vi "S4GUI_003.vi"(7 "Tab ObsEng":enum32{"Obs", "CCD modes", "Guider", "Eng"}(tab)) -> ()   [LabVIEW 2018] (continued)
                n2221 = call-dynamic "Get CCD_Config.vi"("error in (no error)"=w4421, "Interface in"=w4422) -> ("error out"=w4419:errorcluster, "output cluster"=w4418:T31, "Interface out"=w4423:refnum<class "Interface.lvclass">)  [unwired: 7 in]
                n2222 = Bundle By Name(cluster=w4418, "TRIGGER_MODE"=w4406) -> (w4420:T31)
                n2223 = call-dynamic "Set CCD_Config.vi"("error in (no error)"=w4419, "input cluster"=w4420, "Interface in"=w4423) -> ("error out"=w4417:errorcluster, "Interface out"=w4424:refnum<class "Interface.lvclass">)  [unwired: 7 in]
                n2224 = Flatten To String(anything=w4420, error in (no error)=w4417) -> (data string=w4415:string, error out=w4416:errorcluster)  [unwired: 2 in, 1 out]
                n2225 = call "Write flatted cluster.vi"("error in (no error)"=w4416, "flatted cluster"=w4415, "Interface in"=w4424) -> ("error out"=w4426:errorcluster, "Interface out"=w4425:refnum<class "Interface.lvclass">)  [unwired: 7 in]
                n2226 = call-dynamic "Write Interface.vi"("error in (no error)"=w4426, "Interface.lvclass"=w4425, "Channel in"=w4411) -> ("error out"=w4432:errorcluster, "Channel out"=w4433:refnum<class "Channel.lvclass">)  [unwired: 7 in]
                n2227 = call "Write section_name.vi"("error in (no error)"=w4432, "section_name"="CCD_ACS3", "Channel in"=w4433) -> ("error out"=w4430:errorcluster, "Channel out"=w4436:refnum<class "Channel.lvclass">)  [unwired: 7 in]
                n2228 = call-dynamic "save config.vi"("error in (no error)"=w4430, "file config"="lastsaved.cfg", "Channel in"=w4436) -> ("error out"=w4431:errorcluster, "Channel out"=w4437:refnum<class "Channel.lvclass">)  [unwired: 7 in]
                n2229 = call-dynamic "Read State Machine.vi"("error in (no error)"=w4431, "Device in"=w4437) -> ("error out"=w4427:errorcluster, "State Machine.lvclass"=w4439:refnum<class "State Machine.lvclass">, "Device out"=w4438:refnum<class "Channel.lvclass">)  [unwired: 7 in]
                n2230 = call-dynamic "Write State.vi"("error in (no error)"=w4427, "State"=60, "State Machine in"=w4439) -> ("error out"=w4428:errorcluster, "State Machine out"=w4440:refnum<class "State Machine.lvclass">)  [unwired: 7 in]
                n2231 = call-dynamic "Write State Machine.vi"("error in (no error)"=w4428, "State Machine.lvclass"=w4440, "Device in"=w4438) -> ("error out"=w4404:errorcluster, "Device out"=w4405:refnum<class "Channel.lvclass">)  [unwired: 7 in]
                n2232 = call-dynamic "Read prev ciclos.vi"("error in (no error)"=w4404, "Channel in"=w4405) -> ("error out"=w4402:errorcluster, "prev ciclos"=w4400:u32, "Channel out"=w4403:refnum<class "Channel.lvclass">)  [unwired: 7 in]
                n2233 = local write "#cycles ch3"(w4400) -> ()
                n2234 = property on="Cycles Done ch3" class="Slide (strict)"("Scale.Maximum"=w4400, "Scale.Minimum"=0.0 ("Scale.Range:Minimum")) -> ()  [unwired: 2 in, 2 out]
                n2235 = call-dynamic "Write Channel.vi"("error in (no error)"=w4402, "Channel.lvclass"=w4403, "Acquisition in"=w4412) -> ("error out"=w4407:errorcluster, "Acquisition out"=w4408:refnum<class "Acquisition.lvclass">)  [unwired: 7 in]
              }
            }
            n2236 = case shown="True" w4337 {
              tunnel: w4339 -> [w4356 w4367]
              tunnel: w4338 -> [w4355 w4366]
              tunnel: [w4356 w4365] -> w4310
              tunnel: [w4355 w4364] -> w4309
              tunnel: w4307 -> [_ w4363]
              frame False {
              }
              frame True {
                # "nome do arquivo .cfg"
                # "seção no arquivo .cfg"
                n2237 = call-dynamic "Read Channel.vi"("error in (no error)"=w4366, "Acquisition in"=w4367) -> ("error out"=w4394:errorcluster, "Channel.lvclass"=w4395:refnum<class "Channel.lvclass">, "Acquisition out"=w4396:refnum<class "Acquisition.lvclass">)  [unwired: 7 in]
                n2238 = call-dynamic "Read Interface.vi"("error in (no error)"=w4394, "Channel in"=w4395) -> ("error out"=w4387:errorcluster, "Interface.lvclass"=w4386:refnum<class "Interface.lvclass">, "Channel out"=w4397:refnum<class "Channel.lvclass">)  [unwired: 7 in]
                n2239 = call-dynamic "Get CCD_Config.vi"("error in (no error)"=w4387, "Interface in"=w4386) -> ("error out"=w4389:errorcluster, "output cluster"=w4390:T31, "Interface out"=w4385:refnum<class "Interface.lvclass">)  [unwired: 7 in]
                n2240 = Bundle By Name(cluster=w4390, "TRIGGER_MODE"=w4363) -> (w4388:T31)
                n2241 = call-dynamic "Set CCD_Config.vi"("error in (no error)"=w4389, "input cluster"=w4388, "Interface in"=w4385) -> ("error out"=w4391:errorcluster, "Interface out"=w4384:refnum<class "Interface.lvclass">)  [unwired: 7 in]
                n2242 = Flatten To String(anything=w4388, error in (no error)=w4391) -> (data string=w4393:string, error out=w4392:errorcluster)  [unwired: 2 in, 1 out]
                n2243 = call "Write flatted cluster.vi"("error in (no error)"=w4392, "flatted cluster"=w4393, "Interface in"=w4384) -> ("error out"=w4382:errorcluster, "Interface out"=w4383:refnum<class "Interface.lvclass">)  [unwired: 7 in]
                n2244 = call-dynamic "Write Interface.vi"("error in (no error)"=w4382, "Interface.lvclass"=w4383, "Channel in"=w4397) -> ("error out"=w4376:errorcluster, "Channel out"=w4375:refnum<class "Channel.lvclass">)  [unwired: 7 in]
                n2245 = call "Write section_name.vi"("error in (no error)"=w4376, "section_name"="CCD_ACS4", "Channel in"=w4375) -> ("error out"=w4378:errorcluster, "Channel out"=w4372:refnum<class "Channel.lvclass">)  [unwired: 7 in]
                n2246 = call-dynamic "save config.vi"("error in (no error)"=w4378, "file config"="lastsaved.cfg", "Channel in"=w4372) -> ("error out"=w4377:errorcluster, "Channel out"=w4371:refnum<class "Channel.lvclass">)  [unwired: 7 in]
                n2247 = call-dynamic "Read State Machine.vi"("error in (no error)"=w4377, "Device in"=w4371) -> ("error out"=w4381:errorcluster, "State Machine.lvclass"=w4369:refnum<class "State Machine.lvclass">, "Device out"=w4370:refnum<class "Channel.lvclass">)  [unwired: 7 in]
                n2248 = call-dynamic "Write State.vi"("error in (no error)"=w4381, "State"=60, "State Machine in"=w4369) -> ("error out"=w4380:errorcluster, "State Machine out"=w4368:refnum<class "State Machine.lvclass">)  [unwired: 7 in]
                n2249 = call-dynamic "Write State Machine.vi"("error in (no error)"=w4380, "State Machine.lvclass"=w4368, "Device in"=w4370) -> ("error out"=w4361:errorcluster, "Device out"=w4362:refnum<class "Channel.lvclass">)  [unwired: 7 in]
                n2250 = call-dynamic "Read prev ciclos.vi"("error in (no error)"=w4361, "Channel in"=w4362) -> ("error out"=w4359:errorcluster, "prev ciclos"=w4357:u32, "Channel out"=w4360:refnum<class "Channel.lvclass">)  [unwired: 7 in]
                n2251 = local write "#cycles ch4"(w4357) -> ()
                n2252 = property on="Cycles Done ch4" class="Slide (strict)"("Scale.Maximum"=w4357, "Scale.Minimum"=0.0 ("Scale.Range:Minimum")) -> ()  [unwired: 2 in, 2 out]
                n2253 = call-dynamic "Write Channel.vi"("error in (no error)"=w4359, "Channel.lvclass"=w4360, "Acquisition in"=w4396) -> ("error out"=w4364:errorcluster, "Acquisition out"=w4365:refnum<class "Acquisition.lvclass">)  [unwired: 7 in]
              }
            }
            n2254 = case shown="True" w4343 {
              tunnel: w4345 -> [w4442 w4453]
              tunnel: w4344 -> [w4441 w4452]
              tunnel: [w4442 w4451] -> w4314
              tunnel: [w4441 w4450] -> w4313
              tunnel: w4307 -> [_ w4449]
              frame False {
              }
              frame True {
                # "nome do arquivo .cfg"
                # "seção no arquivo .cfg"
                n2255 = call-dynamic "Read Channel.vi"("error in (no error)"=w4452, "Acquisition in"=w4453) -> ("error out"=w4457:errorcluster, "Channel.lvclass"=w4456:refnum<class "Channel.lvclass">, "Acquisition out"=w4455:refnum<class "Acquisition.lvclass">)  [unwired: 7 in]
                n2256 = call-dynamic "Read Interface.vi"("error in (no error)"=w4457, "Channel in"=w4456) -> ("error out"=w4464:errorcluster, "Interface.lvclass"=w4465:refnum<class "Interface.lvclass">, "Channel out"=w4454:refnum<class "Channel.lvclass">)  [unwired: 7 in]
                n2257 = call-dynamic "Get CCD_Config.vi"("error in (no error)"=w4464, "Interface in"=w4465) -> ("error out"=w4462:errorcluster, "output cluster"=w4461:T31, "Interface out"=w4466:refnum<class "Interface.lvclass">)  [unwired: 7 in]
                n2258 = Bundle By Name(cluster=w4461, "TRIGGER_MODE"=w4449) -> (w4463:T31)
                n2259 = call-dynamic "Set CCD_Config.vi"("error in (no error)"=w4462, "input cluster"=w4463, "Interface in"=w4466) -> ("error out"=w4460:errorcluster, "Interface out"=w4467:refnum<class "Interface.lvclass">)  [unwired: 7 in]
                n2260 = Flatten To String(anything=w4463, error in (no error)=w4460) -> (data string=w4458:string, error out=w4459:errorcluster)  [unwired: 2 in, 1 out]
                n2261 = call "Write flatted cluster.vi"("error in (no error)"=w4459, "flatted cluster"=w4458, "Interface in"=w4467) -> ("error out"=w4469:errorcluster, "Interface out"=w4468:refnum<class "Interface.lvclass">)  [unwired: 7 in]
                n2262 = call-dynamic "Write Interface.vi"("error in (no error)"=w4469, "Interface.lvclass"=w4468, "Channel in"=w4454) -> ("error out"=w4475:errorcluster, "Channel out"=w4476:refnum<class "Channel.lvclass">)  [unwired: 7 in]
                n2263 = call "Write section_name.vi"("error in (no error)"=w4475, "section_name"="CCD_ACS2", "Channel in"=w4476) -> ("error out"=w4473:errorcluster, "Channel out"=w4479:refnum<class "Channel.lvclass">)  [unwired: 7 in]
                n2264 = call-dynamic "save config.vi"("error in (no error)"=w4473, "file config"="lastsaved.cfg", "Channel in"=w4479) -> ("error out"=w4474:errorcluster, "Channel out"=w4480:refnum<class "Channel.lvclass">)  [unwired: 7 in]
                n2265 = call-dynamic "Read State Machine.vi"("error in (no error)"=w4474, "Device in"=w4480) -> ("error out"=w4470:errorcluster, "State Machine.lvclass"=w4482:refnum<class "State Machine.lvclass">, "Device out"=w4481:refnum<class "Channel.lvclass">)  [unwired: 7 in]
                n2266 = call-dynamic "Write State.vi"("error in (no error)"=w4470, "State"=60, "State Machine in"=w4482) -> ("error out"=w4471:errorcluster, "State Machine out"=w4483:refnum<class "State Machine.lvclass">)  [unwired: 7 in]
                n2267 = call-dynamic "Write State Machine.vi"("error in (no error)"=w4471, "State Machine.lvclass"=w4483, "Device in"=w4481) -> ("error out"=w4447:errorcluster, "Device out"=w4448:refnum<class "Channel.lvclass">)  [unwired: 7 in]
                n2268 = call-dynamic "Read prev ciclos.vi"("error in (no error)"=w4447, "Channel in"=w4448) -> ("error out"=w4445:errorcluster, "prev ciclos"=w4443:u32, "Channel out"=w4446:refnum<class "Channel.lvclass">)  [unwired: 7 in]
                n2269 = local write "#cycles ch2"(w4443) -> ()
                n2270 = property on="Cycles Done ch2" class="Slide (strict)"("Scale.Maximum"=w4443, "Scale.Minimum"=0.0 ("Scale.Range:Minimum")) -> ()  [unwired: 2 in, 2 out]
                n2271 = call-dynamic "Write Channel.vi"("error in (no error)"=w4445, "Channel.lvclass"=w4446, "Acquisition in"=w4455) -> ("error out"=w4450:errorcluster, "Acquisition out"=w4451:refnum<class "Acquisition.lvclass">)  [unwired: 7 in]
              }
            }
            n2272 = case shown="True" w4346 {
              tunnel: [w4484 w4522] -> w4315
              tunnel: [w4485 w4521] -> w4316
              tunnel: w4348 -> [w4485 w4494]
              tunnel: w4347 -> [w4484 w4493]
              tunnel: w4307 -> [_ w4492]
              frame False {
              }
              frame True {
                # "nome do arquivo .cfg"
                # "seção no arquivo .cfg"
                n2273 = call-dynamic "Read Channel.vi"("error in (no error)"=w4493, "Acquisition in"=w4494) -> ("error out"=w4523:errorcluster, "Channel.lvclass"=w4524:refnum<class "Channel.lvclass">, "Acquisition out"=w4525:refnum<class "Acquisition.lvclass">)  [unwired: 7 in]
                n2274 = call-dynamic "Read Interface.vi"("error in (no error)"=w4523, "Channel in"=w4524) -> ("error out"=w4514:errorcluster, "Interface.lvclass"=w4513:refnum<class "Interface.lvclass">, "Channel out"=w4526:refnum<class "Channel.lvclass">)  [unwired: 7 in]
                n2275 = call-dynamic "Get CCD_Config.vi"("error in (no error)"=w4514, "Interface in"=w4513) -> ("error out"=w4516:errorcluster, "output cluster"=w4517:T31, "Interface out"=w4512:refnum<class "Interface.lvclass">)  [unwired: 7 in]
                n2276 = Bundle By Name(cluster=w4517, "TRIGGER_MODE"=w4492) -> (w4515:T31)
                n2277 = call-dynamic "Set CCD_Config.vi"("error in (no error)"=w4516, "input cluster"=w4515, "Interface in"=w4512) -> ("error out"=w4518:errorcluster, "Interface out"=w4511:refnum<class "Interface.lvclass">)  [unwired: 7 in]
                n2278 = Flatten To String(anything=w4515, error in (no error)=w4518) -> (data string=w4520:string, error out=w4519:errorcluster)  [unwired: 2 in, 1 out]
                n2279 = call "Write flatted cluster.vi"("error in (no error)"=w4519, "flatted cluster"=w4520, "Interface in"=w4511) -> ("error out"=w4509:errorcluster, "Interface out"=w4510:refnum<class "Interface.lvclass">)  [unwired: 7 in]
                n2280 = call-dynamic "Write Interface.vi"("error in (no error)"=w4509, "Interface.lvclass"=w4510, "Channel in"=w4526) -> ("error out"=w4504:errorcluster, "Channel out"=w4503:refnum<class "Channel.lvclass">)  [unwired: 7 in]
                n2281 = call "Write section_name.vi"("error in (no error)"=w4504, "section_name"="CCD_ACS1", "Channel in"=w4503) -> ("error out"=w4505:errorcluster, "Channel out"=w4500:refnum<class "Channel.lvclass">)  [unwired: 7 in]
                n2282 = call-dynamic "save config.vi"("error in (no error)"=w4505, "file config"="lastsaved.cfg", "Channel in"=w4500) -> ("error out"=w4495:errorcluster, "Channel out"=w4496:refnum<class "Channel.lvclass">)  [unwired: 7 in]
                n2283 = call-dynamic "Read State Machine.vi"("error in (no error)"=w4495, "Device in"=w4496) -> ("error out"=w4508:errorcluster, "State Machine.lvclass"=w4498:refnum<class "State Machine.lvclass">, "Device out"=w4499:refnum<class "Channel.lvclass">)  [unwired: 7 in]
                n2284 = call-dynamic "Write State.vi"("error in (no error)"=w4508, "State"=60, "State Machine in"=w4498) -> ("error out"=w4507:errorcluster, "State Machine out"=w4497:refnum<class "State Machine.lvclass">)  [unwired: 7 in]
                n2285 = call-dynamic "Write State Machine.vi"("error in (no error)"=w4507, "State Machine.lvclass"=w4497, "Device in"=w4499) -> ("error out"=w4490:errorcluster, "Device out"=w4491:refnum<class "Channel.lvclass">)  [unwired: 7 in]
                n2286 = call-dynamic "Read prev ciclos.vi"("error in (no error)"=w4490, "Channel in"=w4491) -> ("error out"=w4488:errorcluster, "prev ciclos"=w4486:u32, "Channel out"=w4489:refnum<class "Channel.lvclass">)  [unwired: 7 in]
                n2287 = local write "#cycles ch1"(w4486) -> ()
                n2288 = property on="Cycles Done ch1" class="Slide (strict)"("Scale.Maximum"=w4486, "Scale.Minimum"=0.0 ("Scale.Range:Minimum")) -> ()  [unwired: 2 in, 2 out]
                n2289 = call-dynamic "Write Channel.vi"("error in (no error)"=w4488, "Channel.lvclass"=w4489, "Acquisition in"=w4525) -> ("error out"=w4522:errorcluster, "Acquisition out"=w4521:refnum<class "Acquisition.lvclass">)  [unwired: 7 in]
              }
            }
            n2290 = call-dynamic "Write AcquisitionA.vi"("error in (no error)"=w4315, "Acquisition.lvclass"=w4316, "S4ACS_GUI in"=w4317) -> ("error out"=w4323:errorcluster, "S4ACS_GUI out"=w4326:refnum<class "S4GUI.lvclass">)  [unwired: 7 in]
            n2291 = call "Write AcquisitionB.vi"("error in (no error)"=w4313, "Acquisition.lvclass"=w4314, "S4ACS_GUI in"=w4326) -> ("error out"=w4322:errorcluster, "S4ACS_GUI out"=w4325:refnum<class "S4GUI.lvclass">)  [unwired: 7 in]
            n2292 = call-dynamic "Write AcquisitionC.vi"("error in (no error)"=w4311, "Acquisition.lvclass"=w4312, "S4ACS_GUI in"=w4325) -> ("error out"=w4321:errorcluster, "S4ACS_GUI out"=w4324:refnum<class "S4GUI.lvclass">)  [unwired: 7 in]
            n2293 = call-dynamic "Write AcquisitionD.vi"("error in (no error)"=w4309, "Acquisition.lvclass"=w4310, "S4ACS_GUI in"=w4324) -> ("error out"=w4320:errorcluster, "S4ACS_GUI out"=w4319:refnum<class "S4GUI.lvclass">)  [unwired: 7 in]
            n2294 = Merge Errors(w4323, w4322, w4321, w4320) -> (w4318:errorcluster)
          }
        }
        n2295 = Concatenate Strings(w4071, " MODE SELECTED" ("User Event")) -> (w4076:string)
        n2296 = call-dynamic "Write sync.vi"("error in (no error)"=w4089, "sync"=w4091, "S4ACS_GUI in"=w4090) -> ("error out"=w4074:errorcluster, "S4ACS_GUI out"=w4075:refnum<class "S4GUI.lvclass">)  [unwired: 7 in]
        n2297 = call-dynamic "Write User Event.vi"("error in (no error)"=w4074, "User Event"=w4076, "S4GUI in"=w4075) -> ("error out"=w4072:errorcluster, "S4GUI out"=w4073:refnum<class "S4GUI.lvclass">)  [unwired: 7 in]
      }
      event "SendExpose": Value Change {
        n2298 = event-data() -> ("NewVal"=w4527:bool)  [unwired: 1 in]
        n2299 = disable-structure shown="Enabled" {
          disable-tunnel: w4527 -> [w4665 w4666]
          disable-tunnel: [w4664 w4666] -> w4528
          frame Disabled {
            n2300 = Not(x=w4665) -> (.not. x?=w4664:bool)
          }
          frame Enabled {
          }
        }
        n2301 = disable-structure shown="Enabled" {
          disable-tunnel: w4612 -> [w4627 w4663]
          disable-tunnel: w4611 -> [w4618 w4662]
          disable-tunnel: [w4615 w4663] -> w4530
          disable-tunnel: [w4614 w4662] -> w4529
          disable-tunnel: w4527 -> [w4613 _]
          frame Disabled {
            n2302 = call-dynamic "Read Sync Box.lvclass.vi"("error in (no error)"=w4618, "SPARC4_AC in"=w4627) -> ("error out"=w4620:errorcluster, "Sync Box.lvclass"=w4626:refnum<class "Sync Box.lvclass">, "SPARC4_AC out"=w4623:refnum<class "S4GUI.lvclass">)  [unwired: 7 in]
            n2303 = call-dynamic "Read Stream.vi"("error in (no error)"=w4620, "Server in"=w4626) -> ("error out"=w4619:errorcluster, "Stream.lvclass"=w4628:refnum<class "Stream.lvclass">, "Server out"=w4617:refnum<class "Sync Box.lvclass">)  [unwired: 7 in]
            n2304 = case shown="True" w4613 {
              tunnel: [w4631 w4648] -> w4621
              tunnel: w4628 -> [w4633 w4638]
              tunnel: [w4632 w4644] -> w4625
              tunnel: w4619 -> [w4630 w4636]
              tunnel: w4617 -> [w4629 w4637]
              tunnel: [w4629 w4637] -> w4616
              frame False {
                n2305 = call-dynamic "End.vi"("error in (no error)"=w4630, "Stream in"=w4633) -> ("error out"=w4631:errorcluster, "Stream out"=w4632:refnum<class "Stream.lvclass">)  [unwired: 8 in]
              }
              frame True {
                w4641 = errorcluster {"status"=FALSE, "code"=0, "source"=""} ("error in (no error)")
                w4659 = FALSE ("Wait Until Done")
                w4654 = FALSE ("Wait Until Done")
                n2306 = call-dynamic "Read comfile name1.vi"("error in (no error)"=w4636, "Stream in"=w4638) -> ("error out"=w4650:errorcluster, "comfile name1"=w4651:string, "Stream out"=w4647:refnum<class "Stream.lvclass">)  [unwired: 7 in]
                n2307 = call <vilib>:"Application Directory.vi"() -> ("Application Directory"=w4656:path)
                n2308 = call <vilib>:"Application Directory.vi"() -> ("Application Directory"=w4660:path)
                n2309 = Build Path(base path=w4660, name or relative path=w4651) -> (appended path=w4661:path)
                n2310 = Open VI Reference(vi path=w4661, error in (no error)=w4650) -> (vi reference=w4653:refnum<vi>, error out=w4652:errorcluster)  [unwired: 4 in]
                n2311 = invoke class="VI" method="Run VI"(reference=w4653, error in=w4652, "Wait until done"=w4654, "Auto Dispose Ref"=w4654) -> (reference out=w4643:refnum<vi>, error out=→"error out 7":errorcluster)  [unwired: 1 in, 3 out]
                n2312 = call-dynamic "Write commfile ref1.vi"("error in (no error)"=w4641, "commfile ref1"=w4643, "Stream in"=w4647) -> ("error out"=w4635:errorcluster, "Stream out"=w4646:refnum<class "Stream.lvclass">)  [unwired: 7 in]
                n2313 = call-dynamic "Read comfile name2.vi"("error in (no error)"=w4635, "Stream in"=w4646) -> ("error out"=w4634:errorcluster, "comfile name2"=w4649:string, "Stream out"=w4645:refnum<class "Stream.lvclass">)  [unwired: 7 in]
                n2314 = Build Path(base path=w4656, name or relative path=w4649) -> (appended path=w4655:path)
                n2315 = Open VI Reference(vi path=w4655, error in (no error)=w4634) -> (vi reference=w4657:refnum<vi>, error out=w4658:errorcluster)  [unwired: 4 in]
                n2316 = invoke class="VI" method="Run VI"(reference=w4657, error in=w4658, "Wait until done"=w4659, "Auto Dispose Ref"=w4659) -> (reference out=w4642:refnum<vi>, error out=→"error out 8":errorcluster)  [unwired: 1 in, 3 out]
                n2317 = call-dynamic "Write commfile ref2.vi"("error in (no error)"=w4641, "commfile ref2"=w4642, "Stream in"=w4645) -> ("error out"=w4648:errorcluster, "Stream out"=w4644:refnum<class "Stream.lvclass">)  [unwired: 7 in]
              }
            }
            n2318 = call-dynamic "Write Stream.vi"("error in (no error)"=w4621, "Stream.lvclass"=w4625, "Server in"=w4616) -> ("error out"=w4622:errorcluster, "Server out"=w4624:refnum<class "Sync Box.lvclass">)  [unwired: 7 in]
            n2319 = call-dynamic "Write Sync Box.lvclass.vi"("error in (no error)"=w4622, "Sync Box.lvclass"=w4624, "SPARC4_AC in"=w4623) -> ("error out"=w4614:errorcluster, "SPARC4_AC out"=w4615:refnum<class "S4GUI.lvclass">)  [unwired: 7 in]
          }
          frame Enabled {
          }
        }
        n2320 = call-dynamic "Read AcquisitionC.vi"("error in (no error)"=w4529, "S4ACS_GUI in"=w4530) -> ("error out"=w4554:errorcluster, "Acquisition.lvclass"=w4555:refnum<class "Acquisition.lvclass">)  [unwired: 7 in, 1 out]
        n2321 = call-dynamic "Read AcquisitionA.vi"("error in (no error)"=w4529, "S4ACS_GUI in"=w4530) -> ("error out"=w4591:errorcluster, "Acquisition.lvclass"=w4590:refnum<class "Acquisition.lvclass">, "S4ACS_GUI out"=w4607:refnum<class "S4GUI.lvclass">)  [unwired: 7 in]
        n2322 = call "Read AcquisitionB.vi"("error in (no error)"=w4529, "S4ACS_GUI in"=w4530) -> ("error out"=w4571:errorcluster, "Acquisition.lvclass"=w4572:refnum<class "Acquisition.lvclass">)  [unwired: 7 in, 1 out]
        n2323 = call-dynamic "Read AcquisitionD.vi"("error in (no error)"=w4529, "S4ACS_GUI in"=w4530) -> ("error out"=w4537:errorcluster, "Acquisition.lvclass"=w4538:refnum<class "Acquisition.lvclass">)  [unwired: 7 in, 1 out]
        n2324 = call-dynamic "Read Channel.vi"("error in (no error)"=w4537, "Acquisition in"=w4538) -> ("error out"=w4540:errorcluster, "Channel.lvclass"=w4542:refnum<class "Channel.lvclass">, "Acquisition out"=w4551:refnum<class "Acquisition.lvclass">)  [unwired: 7 in]
        n2325 = call-dynamic "Read Channel.vi"("error in (no error)"=w4554, "Acquisition in"=w4555) -> ("error out"=w4557:errorcluster, "Channel.lvclass"=w4559:refnum<class "Channel.lvclass">, "Acquisition out"=w4568:refnum<class "Acquisition.lvclass">)  [unwired: 7 in]
        n2326 = call-dynamic "Read Channel.vi"("error in (no error)"=w4571, "Acquisition in"=w4572) -> ("error out"=w4574:errorcluster, "Channel.lvclass"=w4576:refnum<class "Channel.lvclass">, "Acquisition out"=w4585:refnum<class "Acquisition.lvclass">)  [unwired: 7 in]
        n2327 = call-dynamic "Read Channel.vi"("error in (no error)"=w4591, "Acquisition in"=w4590) -> ("error out"=w4587:errorcluster, "Channel.lvclass"=w4589:refnum<class "Channel.lvclass">, "Acquisition out"=w4600:refnum<class "Acquisition.lvclass">)  [unwired: 7 in]
        n2328 = call-dynamic "Write wait_expose.vi"("error in (no error)"=w4540, "wait_expose"=w4528, "Channel in"=w4542) -> ("error out"=w4539:errorcluster, "Channel out"=w4541:refnum<class "Channel.lvclass">)  [unwired: 7 in]
        n2329 = call-dynamic "Write wait_expose.vi"("error in (no error)"=w4557, "wait_expose"=w4528, "Channel in"=w4559) -> ("error out"=w4556:errorcluster, "Channel out"=w4558:refnum<class "Channel.lvclass">)  [unwired: 7 in]
        n2330 = call-dynamic "Write wait_expose.vi"("error in (no error)"=w4574, "wait_expose"=w4528, "Channel in"=w4576) -> ("error out"=w4573:errorcluster, "Channel out"=w4575:refnum<class "Channel.lvclass">)  [unwired: 7 in]
        n2331 = call-dynamic "Write wait_expose.vi"("error in (no error)"=w4587, "wait_expose"=w4528, "Channel in"=w4589) -> ("error out"=w4586:errorcluster, "Channel out"=w4588:refnum<class "Channel.lvclass">)  [unwired: 7 in]
        n2332 = call-dynamic "Read State Machine.vi"("error in (no error)"=w4539, "Device in"=w4541) -> ("error out"=w4550:errorcluster, "State Machine.lvclass"=w4546:refnum<class "State Machine.lvclass">, "Device out"=w4547:refnum<class "Channel.lvclass">)  [unwired: 7 in]
        n2333 = call-dynamic "Read State Machine.vi"("error in (no error)"=w4556, "Device in"=w4558) -> ("error out"=w4567:errorcluster, "State Machine.lvclass"=w4563:refnum<class "State Machine.lvclass">, "Device out"=w4564:refnum<class "Channel.lvclass">)  [unwired: 7 in]
        n2334 = call-dynamic "Read State Machine.vi"("error in (no error)"=w4573, "Device in"=w4575) -> ("error out"=w4584:errorcluster, "State Machine.lvclass"=w4580:refnum<class "State Machine.lvclass">, "Device out"=w4581:refnum<class "Channel.lvclass">)  [unwired: 7 in]
        n2335 = call-dynamic "Read State Machine.vi"("error in (no error)"=w4586, "Device in"=w4588) -> ("error out"=w4599:errorcluster, "State Machine.lvclass"=w4595:refnum<class "State Machine.lvclass">, "Device out"=w4596:refnum<class "Channel.lvclass">)  [unwired: 7 in]
        n2336 = call-dynamic "Write State.vi"("error in (no error)"=w4550, "State"=40, "State Machine in"=w4546) -> ("error out"=w4549:errorcluster, "State Machine out"=w4545:refnum<class "State Machine.lvclass">)  [unwired: 7 in]
        n2337 = call-dynamic "Write State.vi"("error in (no error)"=w4567, "State"=40, "State Machine in"=w4563) -> ("error out"=w4566:errorcluster, "State Machine out"=w4562:refnum<class "State Machine.lvclass">)  [unwired: 7 in]
        n2338 = call-dynamic "Write State.vi"("error in (no error)"=w4584, "State"=40, "State Machine in"=w4580) -> ("error out"=w4583:errorcluster, "State Machine out"=w4579:refnum<class "State Machine.lvclass">)  [unwired: 7 in]
        n2339 = call-dynamic "Write State.vi"("error in (no error)"=w4599, "State"=40, "State Machine in"=w4595) -> ("error out"=w4598:errorcluster, "State Machine out"=w4594:refnum<class "State Machine.lvclass">)  [unwired: 7 in]
        n2340 = call-dynamic "Write State Machine.vi"("error in (no error)"=w4549, "State Machine.lvclass"=w4545, "Device in"=w4547) -> ("error out"=w4543:errorcluster, "Device out"=w4544:refnum<class "Channel.lvclass">)  [unwired: 7 in]
        n2341 = call-dynamic "Write State Machine.vi"("error in (no error)"=w4566, "State Machine.lvclass"=w4562, "Device in"=w4564) -> ("error out"=w4560:errorcluster, "Device out"=w4561:refnum<class "Channel.lvclass">)  [unwired: 7 in]
        n2342 = call-dynamic "Write State Machine.vi"("error in (no error)"=w4583, "State Machine.lvclass"=w4579, "Device in"=w4581) -> ("error out"=w4577:errorcluster, "Device out"=w4578:refnum<class "Channel.lvclass">)  [unwired: 7 in]
        n2343 = call-dynamic "Write State Machine.vi"("error in (no error)"=w4598, "State Machine.lvclass"=w4594, "Device in"=w4596) -> ("error out"=w4592:errorcluster, "Device out"=w4593:refnum<class "Channel.lvclass">)  [unwired: 7 in]
        n2344 = call-dynamic "Write Channel.vi"("error in (no error)"=w4543, "Channel.lvclass"=w4544, "Acquisition in"=w4551) -> ("error out"=w4535:errorcluster, "Acquisition out"=w4536:refnum<class "Acquisition.lvclass">)  [unwired: 7 in]
        n2345 = call-dynamic "Write Channel.vi"("error in (no error)"=w4560, "Channel.lvclass"=w4561, "Acquisition in"=w4568) -> ("error out"=w4553:errorcluster, "Acquisition out"=w4552:refnum<class "Acquisition.lvclass">)  [unwired: 7 in]
        n2346 = call-dynamic "Write Channel.vi"("error in (no error)"=w4577, "Channel.lvclass"=w4578, "Acquisition in"=w4585) -> ("error out"=w4570:errorcluster, "Acquisition out"=w4569:refnum<class "Acquisition.lvclass">)  [unwired: 7 in]
        n2347 = call-dynamic "Write Channel.vi"("error in (no error)"=w4592, "Channel.lvclass"=w4593, "Acquisition in"=w4600) -> ("error out"=w4605:errorcluster, "Acquisition out"=w4606:refnum<class "Acquisition.lvclass">)  [unwired: 7 in]
        n2348 = call-dynamic "Write AcquisitionA.vi"("error in (no error)"=w4605, "Acquisition.lvclass"=w4606, "S4ACS_GUI in"=w4607) -> ("error out"=w4604:errorcluster, "S4ACS_GUI out"=w4610:refnum<class "S4GUI.lvclass">)  [unwired: 7 in]
        n2349 = call "Write AcquisitionB.vi"("error in (no error)"=w4570, "Acquisition.lvclass"=w4569, "S4ACS_GUI in"=w4610) -> ("error out"=w4603:errorcluster, "S4ACS_GUI out"=w4609:refnum<class "S4GUI.lvclass">)  [unwired: 7 in]
        n2350 = call-dynamic "Write AcquisitionC.vi"("error in (no error)"=w4553, "Acquisition.lvclass"=w4552, "S4ACS_GUI in"=w4609) -> ("error out"=w4602:errorcluster, "S4ACS_GUI out"=w4608:refnum<class "S4GUI.lvclass">)  [unwired: 7 in]
        n2351 = call-dynamic "Write AcquisitionD.vi"("error in (no error)"=w4535, "Acquisition.lvclass"=w4536, "S4ACS_GUI in"=w4608) -> ("error out"=w4601:errorcluster, "S4ACS_GUI out"=w4534:refnum<class "S4GUI.lvclass">)  [unwired: 7 in]
        n2352 = Merge Errors(w4604, w4603, w4602, w4601) -> (w4533:errorcluster)
        n2353 = call-dynamic "Write mode EXPOSE.vi"("error in (no error)"=w4533, "mode EXPOSE"=w4528, "S4GUI in"=w4534) -> ("error out"=w4531:errorcluster, "S4GUI out"=w4532:refnum<class "S4GUI.lvclass">)  [unwired: 7 in]
      }
      event "CH1on": Value Change {
        n2354 = event-data() -> ("NewVal"=w4676:bool)  [unwired: 1 in]
        n2355 = call-dynamic "Read AcquisitionA.vi"("error in (no error)"=w4690, "S4ACS_GUI in"=w4691) -> ("error out"=w4682:errorcluster, "Acquisition.lvclass"=w4687:refnum<class "Acquisition.lvclass">, "S4ACS_GUI out"=w4683:refnum<class "S4GUI.lvclass">)  [unwired: 7 in]
        n2356 = call-dynamic "Read Channel.vi"("error in (no error)"=w4682, "Acquisition in"=w4687) -> ("error out"=w4681:errorcluster, "Channel.lvclass"=w4672:refnum<class "Channel.lvclass">, "Acquisition out"=w4686:refnum<class "Acquisition.lvclass">)  [unwired: 7 in]
        n2357 = call-dynamic "Read Stream.vi"("error in (no error)"=w4681, "Server in"=w4686) -> ("error out"=w4674:errorcluster, "Stream.lvclass"=w4675:refnum<class "Stream.lvclass">, "Server out"=w4673:refnum<class "Acquisition.lvclass">)  [unwired: 7 in]
        n2358 = case shown="False" w4676 {
          selector: w4676 -> [w4692 w4714]
          tunnel: [w4698 w4718] -> w4670
          tunnel: w4675 -> [w4707 _]
          tunnel: [w4706 w4721] -> w4669
          tunnel: w4674 -> [w4693 w4715]
          tunnel: w4673 -> [w4694 w4716]
          tunnel: [w4694 w4720] -> w4668
          tunnel: w4672 -> [w4705 w4717]
          tunnel: [w4703 w4717] -> w4667
          tunnel: [w4692 w4714] -> w4671
          frame False {
            # "força FALSE nos parametros do CCD"
            n2359 = call-dynamic "Read Interface.vi"("error in (no error)"=w4693, "Channel in"=w4705) -> ("error out"=w4702:errorcluster, "Interface.lvclass"=w4696:refnum<class "Interface.lvclass">, "Channel out"=w4704:refnum<class "Channel.lvclass">)  [unwired: 7 in]
            n2360 = disable-structure shown="Enabled" {
              disable-tunnel: w4707 -> [w4711 w4713]
              disable-tunnel: [w4710 w4713] -> w4706
              disable-tunnel: [w4709 w4712] -> w4699
              disable-tunnel: w4693 -> [w4708 w4712]
              frame Disabled {
                n2361 = call-dynamic "End.vi"("error in (no error)"=w4708, "Stream in"=w4711) -> ("error out"=w4709:errorcluster, "Stream out"=w4710:refnum<class "Stream.lvclass">)  [unwired: 8 in]
              }
              frame Enabled {
              }
            }
            n2362 = call "Write Checked Params.vi"("error in (no error)"=w4702, "Checked Params"=T14 {"ACQUISITION_MODE"=FALSE, "TRIGGER_MODE"=FALSE, "READ_MODE"=FALSE, "PREAMP"=FALSE, "READOUT_RATE"=FALSE, "VERTICAL_SHIFT_SPEED"=FALSE, "EM_MODE"=FALSE, "EM_GAIN"=FALSE, "SHUTTER_MODE"=FALSE, "SHUTTER_TTL"=FALSE, "SHUTTER_OPENING_TIME"=FALSE, "SHUTTER_CLOSING_TIME"=FALSE, "VBIN"=FALSE, "HBIN"=FALSE, "INITIAL_LINE"=FALSE, "INITIAL_COLUMN"=FALSE, "FINAL_LINE"=FALSE, "FINAL_COLUMN"=FALSE, "FRAME_TRANSFER"=FALSE, "VERTICAL_CLOCK_VOLTAGE"=FALSE, "AD_CHANNEL"=FALSE}, "Interface in"=w4696) -> ("error out"=w4701:errorcluster, "Interface out"=w4695:refnum<class "Interface.lvclass">)  [unwired: 7 in]
            n2363 = call-dynamic "Write Interface.vi"("error in (no error)"=w4701, "Interface.lvclass"=w4695, "Channel in"=w4704) -> ("error out"=w4700:errorcluster, "Channel out"=w4703:refnum<class "Channel.lvclass">)  [unwired: 7 in]
            n2364 = Merge Errors(w4700, w4699) -> (w4698:errorcluster)
          }
          frame True {
            n2365 = call-dynamic "Read Stream.vi"("error in (no error)"=w4715, "Server in"=w4716) -> ("error out"=w4719:errorcluster, "Stream.lvclass"=w4722:refnum<class "Stream.lvclass">, "Server out"=w4720:refnum<class "Acquisition.lvclass">)  [unwired: 7 in]
            n2366 = disable-structure shown="Enabled" {
              disable-tunnel: w4722 -> [w4728 w4738]
              disable-tunnel: [w4727 w4738] -> w4721
              disable-tunnel: w4719 -> [w4725 w4737]
              disable-tunnel: [w4723 w4737] -> w4718
              frame Disabled {
                w4736 = FALSE ("Wait Until Done")
                n2367 = call-dynamic "Read comfile name1.vi"("error in (no error)"=w4725, "Stream in"=w4728) -> ("error out"=w4724:errorcluster, "comfile name1"=w4731:string, "Stream out"=w4726:refnum<class "Stream.lvclass">)  [unwired: 7 in]
                n2368 = call <vilib>:"Application Directory.vi"() -> ("Application Directory"=w4733:path)
                n2369 = Build Path(base path=w4733, name or relative path=w4731) -> (appended path=w4732:path)
                n2370 = Open VI Reference(vi path=w4732, error in (no error)=w4724) -> (vi reference=w4734:refnum<vi>, error out=w4735:errorcluster)  [unwired: 4 in]
                n2371 = invoke class="VI" method="Run VI"(reference=w4734, error in=w4735, "Wait until done"=w4736, "Auto Dispose Ref"=w4736) -> (reference out=w4730:refnum<vi>, error out=w4729:errorcluster)  [unwired: 1 in, 3 out]
                n2372 = call-dynamic "Write commfile ref1.vi"("error in (no error)"=w4729, "commfile ref1"=w4730, "Stream in"=w4726) -> ("error out"=w4723:errorcluster, "Stream out"=w4727:refnum<class "Stream.lvclass">)  [unwired: 7 in]
              }
              frame Enabled {
              }
            }
          }
        }
        n2373 = call-dynamic "Write Stream.vi"("error in (no error)"=w4670, "Stream.lvclass"=w4669, "Server in"=w4668) -> ("error out"=w4680:errorcluster, "Server out"=w4678:refnum<class "Acquisition.lvclass">)  [unwired: 7 in]
        n2374 = call-dynamic "Write enabled.vi"("error in (no error)"=w4680, "enabled"=w4671, "Server in"=w4678) -> ("error out"=w4679:errorcluster, "Server out"=w4677:refnum<class "Acquisition.lvclass">)  [unwired: 7 in]
        n2375 = call-dynamic "Write Channel.vi"("error in (no error)"=w4679, "Channel.lvclass"=w4667, "Acquisition in"=w4677) -> ("error out"=w4685:errorcluster, "Acquisition out"=w4684:refnum<class "Acquisition.lvclass">)  [unwired: 7 in]
        n2376 = call-dynamic "Write AcquisitionA.vi"("error in (no error)"=w4685, "Acquisition.lvclass"=w4684, "S4ACS_GUI in"=w4683) -> ("error out"=w4688:errorcluster, "S4ACS_GUI out"=w4689:refnum<class "S4GUI.lvclass">)  [unwired: 7 in]
      }
      event "CH2on": Value Change {
        n2377 = event-data() -> ("NewVal"=w4740:bool)  [unwired: 1 in]
        n2378 = call "Read AcquisitionB.vi"("error in (no error)"=w4762, "S4ACS_GUI in"=w4763) -> ("error out"=w4754:errorcluster, "Acquisition.lvclass"=w4759:refnum<class "Acquisition.lvclass">, "S4ACS_GUI out"=w4755:refnum<class "S4GUI.lvclass">)  [unwired: 7 in]
        n2379 = call-dynamic "Read Channel.vi"("error in (no error)"=w4754, "Acquisition in"=w4759) -> ("error out"=w4753:errorcluster, "Channel.lvclass"=w4748:refnum<class "Channel.lvclass">, "Acquisition out"=w4758:refnum<class "Acquisition.lvclass">)  [unwired: 7 in]
        n2380 = call-dynamic "Read Stream.vi"("error in (no error)"=w4753, "Server in"=w4758) -> ("error out"=w4744:errorcluster, "Stream.lvclass"=w4741:refnum<class "Stream.lvclass">, "Server out"=w4746:refnum<class "Acquisition.lvclass">)  [unwired: 7 in]
        n2381 = case shown="False" w4740 {
          selector: w4740 -> [w4764 w4786]
          tunnel: [w4770 w4790] -> w4743
          tunnel: w4741 -> [w4779 _]
          tunnel: [w4778 w4793] -> w4742
          tunnel: w4744 -> [w4765 w4787]
          tunnel: w4746 -> [w4766 w4788]
          tunnel: [w4766 w4792] -> w4745
          tunnel: w4748 -> [w4777 w4789]
          tunnel: [w4775 w4789] -> w4747
          tunnel: [w4764 w4786] -> w4739
          frame False {
            # "força FALSE nos parametros do CCD"
            n2382 = call-dynamic "Read Interface.vi"("error in (no error)"=w4765, "Channel in"=w4777) -> ("error out"=w4774:errorcluster, "Interface.lvclass"=w4768:refnum<class "Interface.lvclass">, "Channel out"=w4776:refnum<class "Channel.lvclass">)  [unwired: 7 in]
            n2383 = disable-structure shown="Enabled" {
              disable-tunnel: w4779 -> [w4783 w4785]
              disable-tunnel: [w4782 w4785] -> w4778
              disable-tunnel: [w4781 w4784] -> w4771
              disable-tunnel: w4765 -> [w4780 w4784]
              frame Disabled {
                n2384 = call-dynamic "End.vi"("error in (no error)"=w4780, "Stream in"=w4783) -> ("error out"=w4781:errorcluster, "Stream out"=w4782:refnum<class "Stream.lvclass">)  [unwired: 8 in]
              }
              frame Enabled {
              }
            }
            n2385 = call "Write Checked Params.vi"("error in (no error)"=w4774, "Checked Params"=T14 {"ACQUISITION_MODE"=FALSE, "TRIGGER_MODE"=FALSE, "READ_MODE"=FALSE, "PREAMP"=FALSE, "READOUT_RATE"=FALSE, "VERTICAL_SHIFT_SPEED"=FALSE, "EM_MODE"=FALSE, "EM_GAIN"=FALSE, "SHUTTER_MODE"=FALSE, "SHUTTER_TTL"=FALSE, "SHUTTER_OPENING_TIME"=FALSE, "SHUTTER_CLOSING_TIME"=FALSE, "VBIN"=FALSE, "HBIN"=FALSE, "INITIAL_LINE"=FALSE, "INITIAL_COLUMN"=FALSE, "FINAL_LINE"=FALSE, "FINAL_COLUMN"=FALSE, "FRAME_TRANSFER"=FALSE, "VERTICAL_CLOCK_VOLTAGE"=FALSE, "AD_CHANNEL"=FALSE}, "Interface in"=w4768) -> ("error out"=w4773:errorcluster, "Interface out"=w4767:refnum<class "Interface.lvclass">)  [unwired: 7 in]
            n2386 = call-dynamic "Write Interface.vi"("error in (no error)"=w4773, "Interface.lvclass"=w4767, "Channel in"=w4776) -> ("error out"=w4772:errorcluster, "Channel out"=w4775:refnum<class "Channel.lvclass">)  [unwired: 7 in]
            n2387 = Merge Errors(w4772, w4771) -> (w4770:errorcluster)
          }
          frame True {
            n2388 = call-dynamic "Read Stream.vi"("error in (no error)"=w4787, "Server in"=w4788) -> ("error out"=w4791:errorcluster, "Stream.lvclass"=w4794:refnum<class "Stream.lvclass">, "Server out"=w4792:refnum<class "Acquisition.lvclass">)  [unwired: 7 in]
            n2389 = disable-structure shown="Enabled" {
              disable-tunnel: w4794 -> [w4800 w4810]
              disable-tunnel: [w4799 w4810] -> w4793
              disable-tunnel: w4791 -> [w4797 w4809]
              disable-tunnel: [w4795 w4809] -> w4790
              frame Disabled {
                w4808 = FALSE ("Wait Until Done")
                n2390 = call-dynamic "Read comfile name1.vi"("error in (no error)"=w4797, "Stream in"=w4800) -> ("error out"=w4796:errorcluster, "comfile name1"=w4803:string, "Stream out"=w4798:refnum<class "Stream.lvclass">)  [unwired: 7 in]
                n2391 = call <vilib>:"Application Directory.vi"() -> ("Application Directory"=w4805:path)
                n2392 = Build Path(base path=w4805, name or relative path=w4803) -> (appended path=w4804:path)
                n2393 = Open VI Reference(vi path=w4804, error in (no error)=w4796) -> (vi reference=w4806:refnum<vi>, error out=w4807:errorcluster)  [unwired: 4 in]
                n2394 = invoke class="VI" method="Run VI"(reference=w4806, error in=w4807, "Wait until done"=w4808, "Auto Dispose Ref"=w4808) -> (reference out=w4802:refnum<vi>, error out=w4801:errorcluster)  [unwired: 1 in, 3 out]
                n2395 = call-dynamic "Write commfile ref1.vi"("error in (no error)"=w4801, "commfile ref1"=w4802, "Stream in"=w4798) -> ("error out"=w4795:errorcluster, "Stream out"=w4799:refnum<class "Stream.lvclass">)  [unwired: 7 in]
              }
              frame Enabled {
              }
            }
          }
        }
        n2396 = call-dynamic "Write Stream.vi"("error in (no error)"=w4743, "Stream.lvclass"=w4742, "Server in"=w4745) -> ("error out"=w4750:errorcluster, "Server out"=w4752:refnum<class "Acquisition.lvclass">)  [unwired: 7 in]
        n2397 = call-dynamic "Write enabled.vi"("error in (no error)"=w4750, "enabled"=w4739, "Server in"=w4752) -> ("error out"=w4749:errorcluster, "Server out"=w4751:refnum<class "Acquisition.lvclass">)  [unwired: 7 in]
        n2398 = call-dynamic "Write Channel.vi"("error in (no error)"=w4749, "Channel.lvclass"=w4747, "Acquisition in"=w4751) -> ("error out"=w4757:errorcluster, "Acquisition out"=w4756:refnum<class "Acquisition.lvclass">)  [unwired: 7 in]
        n2399 = call "Write AcquisitionB.vi"("error in (no error)"=w4757, "Acquisition.lvclass"=w4756, "S4ACS_GUI in"=w4755) -> ("error out"=w4760:errorcluster, "S4ACS_GUI out"=w4761:refnum<class "S4GUI.lvclass">)  [unwired: 7 in]
      }
      event "CH3 on": Value Change {
        n2400 = event-data() -> ("NewVal"=w4827:bool)  [unwired: 1 in]
        n2401 = call-dynamic "Read AcquisitionC.vi"("error in (no error)"=w4830, "S4ACS_GUI in"=w4834) -> ("error out"=w4819:errorcluster, "Acquisition.lvclass"=w4824:refnum<class "Acquisition.lvclass">, "S4ACS_GUI out"=w4820:refnum<class "S4GUI.lvclass">)  [unwired: 7 in]
        n2402 = call-dynamic "Read Channel.vi"("error in (no error)"=w4819, "Acquisition in"=w4824) -> ("error out"=w4818:errorcluster, "Channel.lvclass"=w4817:refnum<class "Channel.lvclass">, "Acquisition out"=w4823:refnum<class "Acquisition.lvclass">)  [unwired: 7 in]
        n2403 = call-dynamic "Read Stream.vi"("error in (no error)"=w4818, "Server in"=w4823) -> ("error out"=w4831:errorcluster, "Stream.lvclass"=w4835:refnum<class "Stream.lvclass">, "Server out"=w4829:refnum<class "Acquisition.lvclass">)  [unwired: 7 in]
        n2404 = case shown="False" w4827 {
          selector: w4827 -> [w4836 w4858]
          tunnel: [w4842 w4862] -> w4832
          tunnel: w4835 -> [w4851 _]
          tunnel: [w4850 w4865] -> w4833
          tunnel: w4831 -> [w4837 w4859]
          tunnel: w4829 -> [w4838 w4860]
          tunnel: [w4838 w4864] -> w4828
          tunnel: w4817 -> [w4849 w4861]
          tunnel: [w4847 w4861] -> w4816
          tunnel: [w4836 w4858] -> w4811
          frame False {
            # "força FALSE nos parametros do CCD"
            n2405 = call-dynamic "Read Interface.vi"("error in (no error)"=w4837, "Channel in"=w4849) -> ("error out"=w4846:errorcluster, "Interface.lvclass"=w4840:refnum<class "Interface.lvclass">, "Channel out"=w4848:refnum<class "Channel.lvclass">)  [unwired: 7 in]
            n2406 = disable-structure shown="Disabled" {
              disable-tunnel: w4851 -> [w4855 w4857]
              disable-tunnel: [w4854 w4857] -> w4850
              disable-tunnel: [w4853 w4856] -> w4843
              disable-tunnel: w4837 -> [w4852 w4856]
              frame Disabled {
                n2407 = call-dynamic "End.vi"("error in (no error)"=w4852, "Stream in"=w4855) -> ("error out"=w4853:errorcluster, "Stream out"=w4854:refnum<class "Stream.lvclass">)  [unwired: 8 in]
              }
              frame Enabled {
              }
            }
            n2408 = call "Write Checked Params.vi"("error in (no error)"=w4846, "Checked Params"=T14 {"ACQUISITION_MODE"=FALSE, "TRIGGER_MODE"=FALSE, "READ_MODE"=FALSE, "PREAMP"=FALSE, "READOUT_RATE"=FALSE, "VERTICAL_SHIFT_SPEED"=FALSE, "EM_MODE"=FALSE, "EM_GAIN"=FALSE, "SHUTTER_MODE"=FALSE, "SHUTTER_TTL"=FALSE, "SHUTTER_OPENING_TIME"=FALSE, "SHUTTER_CLOSING_TIME"=FALSE, "VBIN"=FALSE, "HBIN"=FALSE, "INITIAL_LINE"=FALSE, "INITIAL_COLUMN"=FALSE, "FINAL_LINE"=FALSE, "FINAL_COLUMN"=FALSE, "FRAME_TRANSFER"=FALSE, "VERTICAL_CLOCK_VOLTAGE"=FALSE, "AD_CHANNEL"=FALSE}, "Interface in"=w4840) -> ("error out"=w4845:errorcluster, "Interface out"=w4839:refnum<class "Interface.lvclass">)  [unwired: 7 in]
            n2409 = call-dynamic "Write Interface.vi"("error in (no error)"=w4845, "Interface.lvclass"=w4839, "Channel in"=w4848) -> ("error out"=w4844:errorcluster, "Channel out"=w4847:refnum<class "Channel.lvclass">)  [unwired: 7 in]
            n2410 = Merge Errors(w4844, w4843) -> (w4842:errorcluster)
          }
          frame True {
            n2411 = call-dynamic "Read Stream.vi"("error in (no error)"=w4859, "Server in"=w4860) -> ("error out"=w4863:errorcluster, "Stream.lvclass"=w4866:refnum<class "Stream.lvclass">, "Server out"=w4864:refnum<class "Acquisition.lvclass">)  [unwired: 7 in]
            n2412 = disable-structure shown="Enabled" {
              disable-tunnel: w4866 -> [w4872 w4882]
              disable-tunnel: [w4871 w4882] -> w4865
              disable-tunnel: w4863 -> [w4869 w4881]
              disable-tunnel: [w4867 w4881] -> w4862
              frame Disabled {
                w4880 = FALSE ("Wait Until Done")
                n2413 = call-dynamic "Read comfile name1.vi"("error in (no error)"=w4869, "Stream in"=w4872) -> ("error out"=w4868:errorcluster, "comfile name1"=w4875:string, "Stream out"=w4870:refnum<class "Stream.lvclass">)  [unwired: 7 in]
                n2414 = call <vilib>:"Application Directory.vi"() -> ("Application Directory"=w4877:path)
                n2415 = Build Path(base path=w4877, name or relative path=w4875) -> (appended path=w4876:path)
                n2416 = Open VI Reference(vi path=w4876, error in (no error)=w4868) -> (vi reference=w4878:refnum<vi>, error out=w4879:errorcluster)  [unwired: 4 in]
                n2417 = invoke class="VI" method="Run VI"(reference=w4878, error in=w4879, "Wait until done"=w4880, "Auto Dispose Ref"=w4880) -> (reference out=w4874:refnum<vi>, error out=w4873:errorcluster)  [unwired: 1 in, 3 out]
                n2418 = call-dynamic "Write commfile ref1.vi"("error in (no error)"=w4873, "commfile ref1"=w4874, "Stream in"=w4870) -> ("error out"=w4867:errorcluster, "Stream out"=w4871:refnum<class "Stream.lvclass">)  [unwired: 7 in]
              }
              frame Enabled {
              }
            }
          }
        }
        n2419 = call-dynamic "Write Stream.vi"("error in (no error)"=w4832, "Stream.lvclass"=w4833, "Server in"=w4828) -> ("error out"=w4814:errorcluster, "Server out"=w4815:refnum<class "Acquisition.lvclass">)  [unwired: 7 in]
        n2420 = call-dynamic "Write enabled.vi"("error in (no error)"=w4814, "enabled"=w4811, "Server in"=w4815) -> ("error out"=w4812:errorcluster, "Server out"=w4813:refnum<class "Acquisition.lvclass">)  [unwired: 7 in]
        n2421 = call-dynamic "Write Channel.vi"("error in (no error)"=w4812, "Channel.lvclass"=w4816, "Acquisition in"=w4813) -> ("error out"=w4822:errorcluster, "Acquisition out"=w4821:refnum<class "Acquisition.lvclass">)  [unwired: 7 in]
        n2422 = call-dynamic "Write AcquisitionC.vi"("error in (no error)"=w4822, "Acquisition.lvclass"=w4821, "S4ACS_GUI in"=w4820) -> ("error out"=w4825:errorcluster, "S4ACS_GUI out"=w4826:refnum<class "S4GUI.lvclass">)  [unwired: 7 in]
      }
      event "CH4 on": Value Change {
        n2423 = event-data() -> ("NewVal"=w4888:bool)  [unwired: 1 in]
        n2424 = call-dynamic "Read AcquisitionD.vi"("error in (no error)"=w4906, "S4ACS_GUI in"=w4907) -> ("error out"=w4898:errorcluster, "Acquisition.lvclass"=w4903:refnum<class "Acquisition.lvclass">, "S4ACS_GUI out"=w4899:refnum<class "S4GUI.lvclass">)  [unwired: 7 in]
        n2425 = call-dynamic "Read Channel.vi"("error in (no error)"=w4898, "Acquisition in"=w4903) -> ("error out"=w4897:errorcluster, "Channel.lvclass"=w4892:refnum<class "Channel.lvclass">, "Acquisition out"=w4902:refnum<class "Acquisition.lvclass">)  [unwired: 7 in]
        n2426 = call-dynamic "Read Stream.vi"("error in (no error)"=w4897, "Server in"=w4902) -> ("error out"=w4890:errorcluster, "Stream.lvclass"=w4889:refnum<class "Stream.lvclass">, "Server out"=w4891:refnum<class "Acquisition.lvclass">)  [unwired: 7 in]
        n2427 = case shown="False" w4888 {
          selector: w4888 -> [w4908 w4930]
          tunnel: [w4914 w4934] -> w4884
          tunnel: w4889 -> [w4923 _]
          tunnel: [w4922 w4937] -> w4885
          tunnel: w4890 -> [w4909 w4931]
          tunnel: w4891 -> [w4910 w4932]
          tunnel: [w4910 w4936] -> w4886
          tunnel: w4892 -> [w4921 w4933]
          tunnel: [w4919 w4933] -> w4887
          tunnel: [w4908 w4930] -> w4883
          frame False {
            # "força FALSE nos parametros do CCD"
            n2428 = call-dynamic "Read Interface.vi"("error in (no error)"=w4909, "Channel in"=w4921) -> ("error out"=w4918:errorcluster, "Interface.lvclass"=w4912:refnum<class "Interface.lvclass">, "Channel out"=w4920:refnum<class "Channel.lvclass">)  [unwired: 7 in]
            n2429 = disable-structure shown="Disabled" {
              disable-tunnel: w4923 -> [w4927 w4929]
              disable-tunnel: [w4926 w4929] -> w4922
              disable-tunnel: [w4925 w4928] -> w4915
              disable-tunnel: w4909 -> [w4924 w4928]
              frame Disabled {
                n2430 = call-dynamic "End.vi"("error in (no error)"=w4924, "Stream in"=w4927) -> ("error out"=w4925:errorcluster, "Stream out"=w4926:refnum<class "Stream.lvclass">)  [unwired: 8 in]
              }
              frame Enabled {
              }
            }
            n2431 = call "Write Checked Params.vi"("error in (no error)"=w4918, "Checked Params"=T14 {"ACQUISITION_MODE"=FALSE, "TRIGGER_MODE"=FALSE, "READ_MODE"=FALSE, "PREAMP"=FALSE, "READOUT_RATE"=FALSE, "VERTICAL_SHIFT_SPEED"=FALSE, "EM_MODE"=FALSE, "EM_GAIN"=FALSE, "SHUTTER_MODE"=FALSE, "SHUTTER_TTL"=FALSE, "SHUTTER_OPENING_TIME"=FALSE, "SHUTTER_CLOSING_TIME"=FALSE, "VBIN"=FALSE, "HBIN"=FALSE, "INITIAL_LINE"=FALSE, "INITIAL_COLUMN"=FALSE, "FINAL_LINE"=FALSE, "FINAL_COLUMN"=FALSE, "FRAME_TRANSFER"=FALSE, "VERTICAL_CLOCK_VOLTAGE"=FALSE, "AD_CHANNEL"=FALSE}, "Interface in"=w4912) -> ("error out"=w4917:errorcluster, "Interface out"=w4911:refnum<class "Interface.lvclass">)  [unwired: 7 in]
            n2432 = call-dynamic "Write Interface.vi"("error in (no error)"=w4917, "Interface.lvclass"=w4911, "Channel in"=w4920) -> ("error out"=w4916:errorcluster, "Channel out"=w4919:refnum<class "Channel.lvclass">)  [unwired: 7 in]
            n2433 = Merge Errors(w4916, w4915) -> (w4914:errorcluster)
          }
          frame True {
            n2434 = call-dynamic "Read Stream.vi"("error in (no error)"=w4931, "Server in"=w4932) -> ("error out"=w4935:errorcluster, "Stream.lvclass"=w4938:refnum<class "Stream.lvclass">, "Server out"=w4936:refnum<class "Acquisition.lvclass">)  [unwired: 7 in]
            n2435 = disable-structure shown="Enabled" {
              disable-tunnel: w4938 -> [w4944 w4954]
              disable-tunnel: [w4943 w4954] -> w4937
              disable-tunnel: w4935 -> [w4941 w4953]
